vi "CheckGameBoardDeadEndCheck.vi"(8 "error in (no error)":errorcluster, 11 "Board in":T1[][](array[typedef])) -> (0 "error out":errorcluster, 2 "Pass":bool, 3 "Board out":T1[][](array[typedef]))   [LabVIEW 2020]
uses:
  TypeDef/tiles-key-trunct.ctl
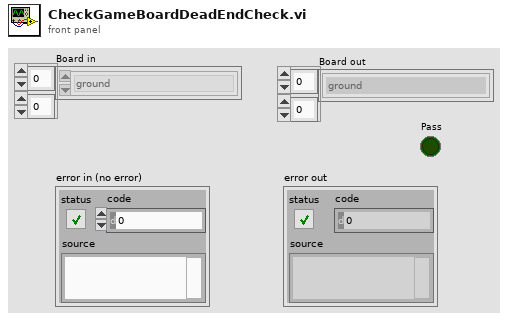
[diagram p1: front panel]
types:
  T1 = typedef "tiles-key-trunct.ctl" = enum16{"ground", "wall", "head (right)", "head (up)", "head (left)", "head (down)", "L-turn (right-up)", "L-turn (up-left)", "L-turn (left-down)", "L-turn (down-right)", "body (right)", "body (up)", "body (left)", "body (down)", "R-turn (right-down)", "R-turn (up-right)", "R-turn (left-up)", "R-turn (down-left)", "tail (right)", "tail (up)", "tail (left)", "tail (down)"}
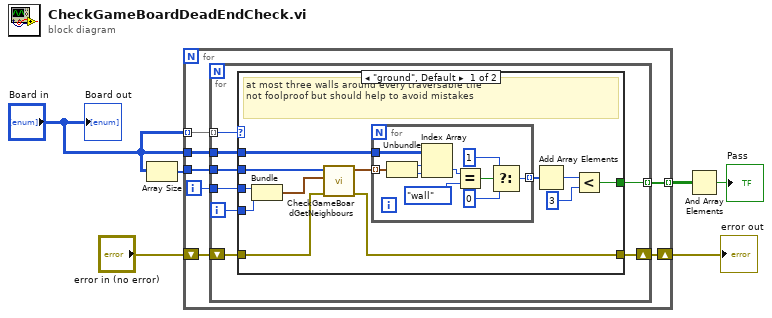
[diagram p0: block diagram]
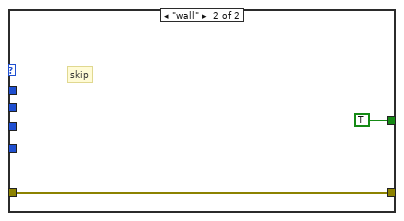
[diagram p2: hidden frame]
diagram:
  n1 = Array Size(array="Board in") -> (size(s)=w6:i32[])
  n2 = for {
    shift-right: [w12] -> w5
    shift-left: "error in (no error)" -> [w13]
    tunnel: w6 -> [w10]
    tunnel: "Board in" -> [w9]
    tunnel: "Board in" -> [w8] mode=indexing
    tunnel: [w7] -> w2 mode=indexing
    i -> [w11]
    n3 = for {
      shift-right: [w20] -> w12
      shift-left: w13 -> [w21]
      tunnel: w11 -> [w19]
      tunnel: w10 -> [w17]
      tunnel: w9 -> [w15]
      tunnel: w8 -> [w16] mode=indexing
      tunnel: [w14] -> w7 mode=indexing
      i -> [w18]
      n4 = case shown="\"ground\", Default" w16 {
        tunnel: w21 -> [w33 w45]
        tunnel: [w32 w45] -> w20
        tunnel: w19 -> [w31 _]
        tunnel: w18 -> [w30 _]
        tunnel: w17 -> [w28 _]
        tunnel: w15 -> [w26 _]
        tunnel: [w22 TRUE] -> w14
        frame "ground", Default {
          # "at most three walls around every traversable tile\nnot foolproof but should help to avoid mistakes"
          n5 = Bundle(w31, w30) -> (w29:cluster{i32, i32})  [unwired: 1 in]
          n6 = call "CheckGameBoardGetNeighbours.vi"("error in (no error)"=w33, "Position in"=w29, "Board size(s)"=w28) -> ("error out"=w32:errorcluster, "Positions out"=w27:cluster{"row":i32, "column":i32}[])  [unwired: 7 in]
          n7 = for {
            tunnel: w27 -> [w43] mode=indexing
            tunnel: w26 -> [w42]
            tunnel: [w34] -> w25 mode=indexing
            n8 = Unbundle(w43) -> ("row"=w41:i32, "column"=w40:i32)
            n9 = Index Array(array=w42, index (row)=w41, index (col)=w40) -> (element=w39:T1)
            n10 = Equal?(x=w39, y=tiles-key-trunct."wall") -> (x = y?=w37:bool)
            n11 = Select(t=1, s=w37, f=0) -> (s? t:f=w34:i32)
          }
          n12 = Add Array Elements(numeric array=w25) -> (sum=w24:i32)
          n13 = Less?(x=w24, y=3) -> (x < y?=w22:bool)
        }
        frame "wall" {
          # "skip"
        }
      }
    }
  }
  "error out" <- w5
  n14 = And Array Elements(Boolean array=w2) -> (logical AND=→"Pass":bool)
  "Board out" <- "Board in"
